vi "Menu Insert.vi"(8 "error in (no error)":errorcluster, 11 "MCLB_Template in":refnum<class "MCLB_Template.lvclass">) -> (0 "error out":errorcluster, 3 "MCLB_Template out":refnum<class "MCLB_Template.lvclass">)   [LabVIEW 2021, in "MCLB_Template.lvclass"]
uses:
  MCLB_Template.lvclass
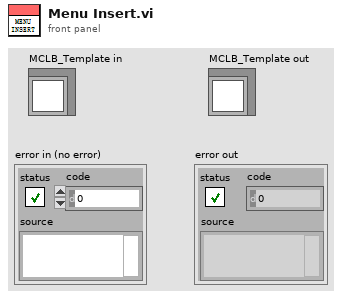
[diagram p1: front panel]
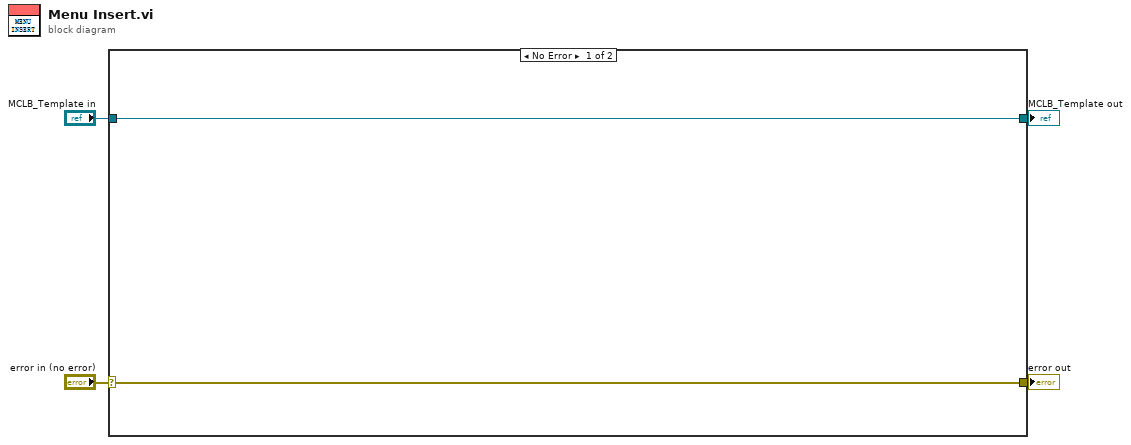
[diagram p0: block diagram]
diagram:
  n1 = case shown="No Error" "error in (no error)" {
    selector: "error in (no error)" -> [w5 w8]
    tunnel: [w5 w8] -> w3
    tunnel: [w6 w7] -> w1
    tunnel: "MCLB_Template in" -> [w6 w7]
    frame No Error {
    }
    frame Error {
    }
  }
  "error out" <- w3
  "MCLB_Template out" <- w1
